vi "SeCrTs-Data transfer_C.vi"(0 "Data FIFO Ref":T1, 3 "error constant":errorcluster) -> (10 "error out":errorcluster)   [LabVIEW 2022 SP3]
uses:
  <vilib>/Platform/TimedLoop/XDataNode/wakeup.ctl
  <vilib>/Platform/TimedLoop/XDataNode/XDNodeRunTimeDep.lvlib
  <vilib>/Platform/TimedLoop/XDataNode/nitl_modes.ctl
  <vilib>/Platform/TimedLoop/XDataNode/timing_clust.ctl
  <vilib>/platform/TimedLoop/XDataNode/XDataNode.xnode
  <resource>/objmgr/ni.dex.rc
  <vilib>/ErrorRing/Error Ring.xnode
  RT Support/SeCrTs-RT_Global_R.vi
  RT Controls/SeCrTs-Data Type Control screen.ctl
  RT Controls/SeCrTs-FGV Read write.ctl
  RT Controls/SeCrTs-Data FIFO.ctl
panel:
  out "Write Backlog":i32
  out "Loop Delay":u32
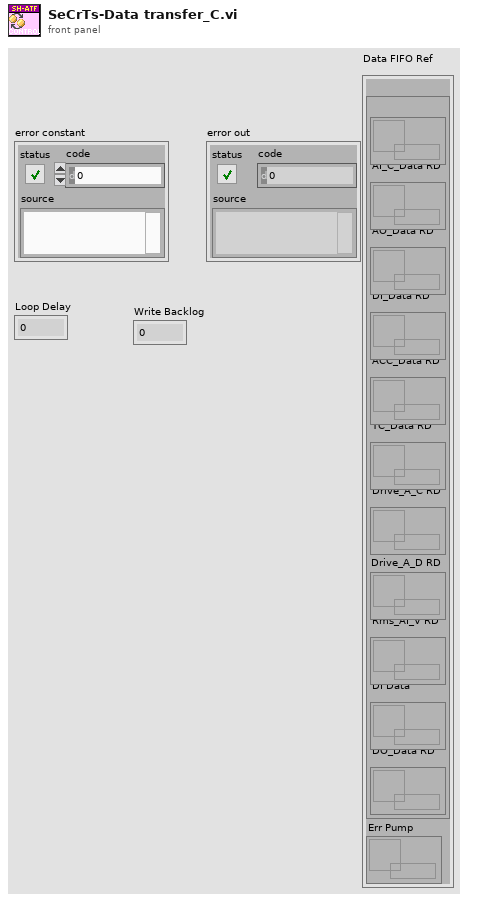
[diagram p1: front panel]
types:
  T1 = typedef "SeCrTs-Data FIFO.ctl" = cluster{"RD":cluster{"AI_V_Data RD":refnum<queue>, "AI_C_Data RD":refnum<queue>, "AO_Data RD":refnum<queue>, "DI_Data RD":refnum<queue>, "ACC_Data RD":refnum<queue>, "TC_Data RD":refnum<queue>, "Drive_A_C RD":refnum<queue>, "Drive_A_D RD":refnum<queue>, "Rms_AI_V RD":refnum<queue>, "DI Data":refnum<queue>, "DO_Data RD":refnum<queue>}, "Err Pump":refnum<queue>}
  T2 = typedef "SeCrTs-FGV Read write.ctl" = enum16{"Write", "Read"}
  T3 = typedef "SeCrTs-Data Type Control screen.ctl" = cluster{"DI_Data":digitalwaveform[], "Drive_A_C":waveform(dbl)[], "Drive_A_D":waveform(dbl)[], "Drive_L_C":waveform(dbl)[], "Drive_L_D":waveform(dbl)[], "Loop Status":bool[], "CDT Timer":dbl, "RT Error":cluster{"Error Code":string, "Error Source":string}, "DO":waveform(dbl)[], "SEQ Monitor":string[], "Device List":string}
  T4 = enum16{"Init", "Read 'All'", "Read 'n'", "Read '1'", "Write '1'", "Write 'n'", "Write 'All'"}
  T5 = typedef "XDNodeRunTimeDep.lvlib/timing_clust.ctl" = cluster{"Expected End [f-1]":u64, "Actual End [f-1]":u64, "Finished Late? [f-1]":bool, "Expected End [i-1]":u64, "Actual End [i-1]":u64, "Finished Late? [i-1]":bool, "Expected Start [i]":u64, "Actual Start [i]":u64, "Expected Start [f]":u64, "Actual Start [f]":u64, "Source Name":string, "Structure Name":string, "Period":i64, "Deadline":i64, "Offset":i64, "Start":i64, "Priority":i32, "Timeout":i32, "Mode":T6, "Wakeup Reason":T7, "Error":errorcluster, "Source Type":string, "Secondary Source Type":string, "Global End Time":u64, "Global Start Time":u64, "Frame Duration":u64, "Iteration Duration":u64, "Assigned CPU":i32, "I/O Scan Engine Mode":u32}
  T6 = typedef "XDNodeRunTimeDep.lvlib/nitl_modes.ctl" = enum32{"No Change", "Process missed periods, maintain original phase", "Discard missed periods, maintain original phase", "Process missed periods, ignore original phase", "Discard missed periods, ignore original phase"}
  T7 = typedef "XDNodeRunTimeDep.lvlib/wakeup.ctl" = enum32{"Normal", "Aborted", "Asynchronous wakeup", "Timing source error", "Timed loop error", "Timeout"}
  T8 = cluster{"Start DAQ":bool, "Stop DAQ":bool, "RT Stop":bool, "RT Exit":bool, "Start Seq":bool}
  T9 = cluster{"Error Code":string, "Error Source":string}
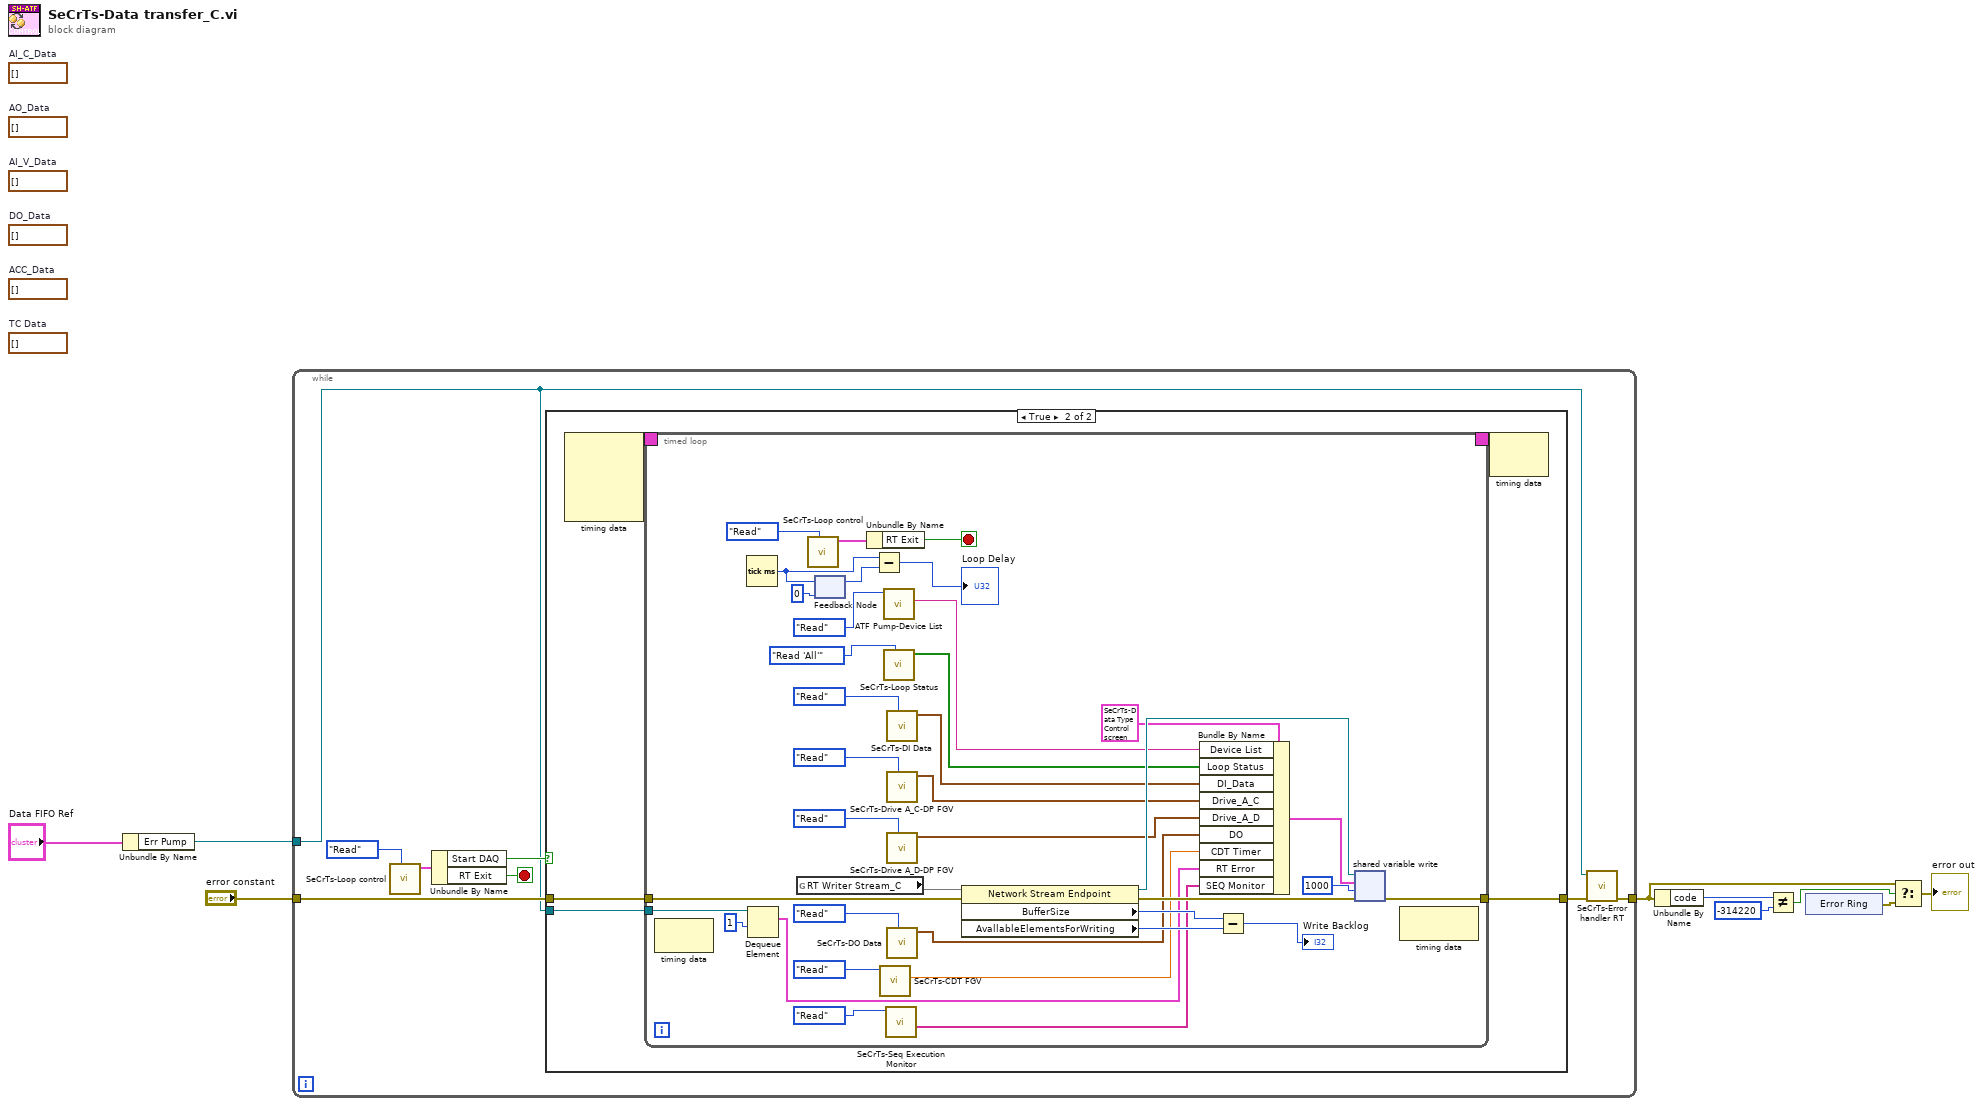
[diagram p0: block diagram]
diagram:
  (unwired) waveform(dbl)[] []  # TC Data
  (unwired) waveform(dbl)[] []  # ACC_Data
  (unwired) waveform(dbl)[] []  # DO_Data
  (unwired) waveform(dbl)[] []  # AO_Data
  (unwired) waveform(dbl)[] []  # AI_C_Data
  (unwired) waveform(dbl)[] []  # AI_V_Data
  n1 = Unbundle By Name("Data FIFO Ref") -> ("Err Pump"=w1:refnum<queue>)
  n2 = while {
    tunnel: "error constant" -> [w17]
    tunnel: [w11] -> w4
    tunnel: w1 -> [w10]
    stop <- w13 stop-if-true
    n3 = call "SeCrTs-Loop control.vi"("Action"=enum16{"Init", "Write", "Read"}."Read") -> ("Loop Control out"=w16:T8)  [unwired: 9 in, 1 out]
    n4 = Unbundle By Name(w16) -> ("Start DAQ"=w14:bool, "RT Exit"=w13:bool)
    n5 = case shown="True" w14 {
      tunnel: w17 -> [w18 w23]
      tunnel: [w18 w22] -> w12
      tunnel: w10 -> [_ w19]
      frame False {
      }
      frame True {
        n6 = node-c288() -> (w21:T5)  [unwired: 4 in]
        n7 = timed-loop {
          tunnel: w23 -> [w54]
          tunnel: [w53] -> w22
          timing: w21 -> [_]
          timing-out: [_] -> w20
          tunnel: w19 -> [w39]
          stop <- w45 stop-if-true
          n8 = node-c288() -> ()  [unwired: 1 in, 1 out]
          n9 = Tick Count (ms)() -> (millisecond timer value=w50:u32)
          n10 = Dequeue Element(queue=w39, timeout in ms (-1)=1) -> (element=w36:T9)  [unwired: 1 in, 3 out]
          n11 = global read "SeCrTs-RT_Global_R.vi" "RT Writer Stream_C"() -> (w48)
          n12 = call "SeCrTs-Loop control.vi"("Action"=enum16{"Init", "Write", "Read"}."Read") -> ("Loop Control out"=w47:T8)  [unwired: 9 in, 1 out]
          n13 = feedback #1(u32 0 ("millisecond timer value")) -> (w51:u32)
          n14 = feedback-in #1(w50) -> ()
          n15 = Unbundle By Name(w47) -> ("RT Exit"=w45:bool)
          n16 = Subtract(x=w50, y=w51) -> (x-y=→"Loop Delay":u32)
          n17 = call "SeCrTs-CDT FGV.vi"("Write/Read"=enum16{"Write", "Read"}."Read") -> ("CDT Out"=w37:dbl)  [unwired: 9 in, 1 out]
          n18 = call "ATF Pump-Device List.vi"("Enum"=enum16{"Write", "Read"}."Read") -> ("DL 2"=w24:string)  [unwired: 9 in, 1 out]
          n19 = call "SeCrTs-Loop Status.vi"("Option"=T4."Read 'All'") -> ("Status List Out"=w43:bool[])  [unwired: 8 in, 2 out]
          n20 = call "SeCrTs-Seq Execution Monitor.vi"("Enum"=enum16{"Read", "Write "}."Read") -> ("Seq Monitor"=w34:string[])  [unwired: 9 in, 1 out]
          n21 = call "SeCrTs-DI Data.vi"("Enum"=enum16{"Write", "Read"}."Read") -> ("Out_DI data"=w32:digitalwaveform[])  [unwired: 10 in]
          n22 = call "SeCrTs-Drive A_C-DP FGV.vi"("Write/Read"=SeCrTs-FGV_Read_write."Read") -> ("Drive A_C  data"=w30:waveform(dbl)[])  [unwired: 9 in, 1 out]
          n23 = call "SeCrTs-Drive A_D-DP FGV.vi"("Write/Read"=SeCrTs-FGV_Read_write."Read") -> ("Drive A_D data"=w28:waveform(dbl)[])  [unwired: 9 in, 1 out]
          n24 = call "SeCrTs-DO Data.vi"("Enum"=enum16{"Write", "Read"}."Read") -> ("out_DO data"=w26:waveform(dbl)[])  [unwired: 10 in]
          n25 = property class="Network Stream Endpoint"(reference=w48, error in=w54) -> (reference out=w59:refnum<k21>, error out=w55:errorcluster, "BufferSize"=w58:i32, "AvallableElementsForWriting"=w57:i32)
          n26 = Bundle By Name(cluster=T3 {"DI_Data"=[], "Drive_A_C"=[], "Drive_A_D"=[], "Drive_L_C"=[], "Drive_L_D"=[], "Loop Status"=[], "CDT Timer"=0.0, "RT Error"={"Error Code"="", "Error Source"=""}, "DO"=[], "SEQ Monitor"=[], "Device List"=""} ("Cluster"), "Device List"=w24, "Loop Status"=w43, "DI_Data"=w32, "Drive_A_C"=w30, "Drive_A_D"=w28, "DO"=w26, "CDT Timer"=w37, "RT Error"=w36, "SEQ Monitor"=w34) -> (w41:T3)
          n27 = Subtract(x=w58, y=w57) -> (x-y=→"Write Backlog":i32)
          n28 = shared-variable-write(w59, w55, w41, 1000 ("timeout ms (-1)")) -> (w53:errorcluster)  [unwired: 2 out]
          n29 = node-c288() -> ()  [unwired: 1 in, 1 out]
        }
        n30 = node-c288(w20) -> ()  [unwired: 1 out]
      }
    }
    n31 = call "SeCrTs-Error handler RT.vi"("error in"=w12, "Message Queue"=w10) -> ("error out"=w11:errorcluster)  [unwired: 8 in, 1 out]
  }
  n32 = Unbundle By Name(w4) -> ("code"=w9:i32)
  n33 = Not Equal?(x=w9, y=-314220) -> (x != y?=w6:bool)
  n34 = xnode "Error Ring"() -> ("error out"=w5:errorcluster)
  n35 = Select(t=w4, s=w6, f=w5) -> (s? t:f=→"error out":errorcluster)
